vi "Send Speed Message_Conti.vi"(6 "Data":u16 format="%x", 8 "Standstill":bool, 9 "Reset":bool) -> (2 "Bit 1 Out":bool, 3 "Bit 0 Out":bool)   [LabVIEW 2015]
uses:
  Protocol State.ctl
  <vilib>/rvi/Emulation/niFpgaSctlEmulationGetInTimedLoop.vi
  <vilib>/rvi/Emulation/niFpgaProcessEmulError.vi
panel:
  out "Timer":u32
  out "Temp Data":u16
  out "State":T1
  out "Bit Count":i32
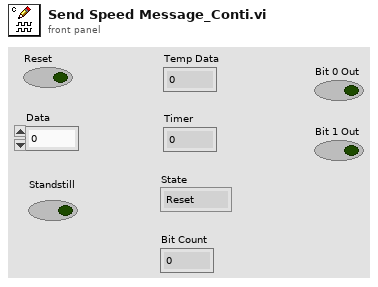
[diagram p1: front panel]
types:
  T1 = typedef "Protocol State.ctl" = enum16{"Reset", "Speed Pulse", "Delay After SP", "DP First Half", "Delay During First Half", "DP Second Half", "Delay During Second Half", "Idle"}
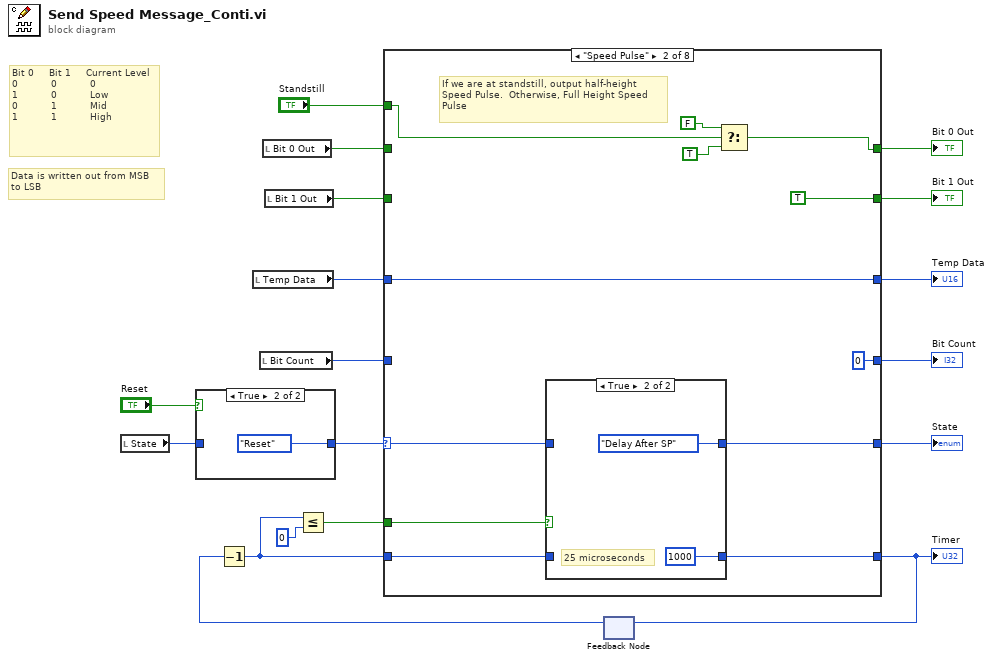
[diagram p0: block diagram]
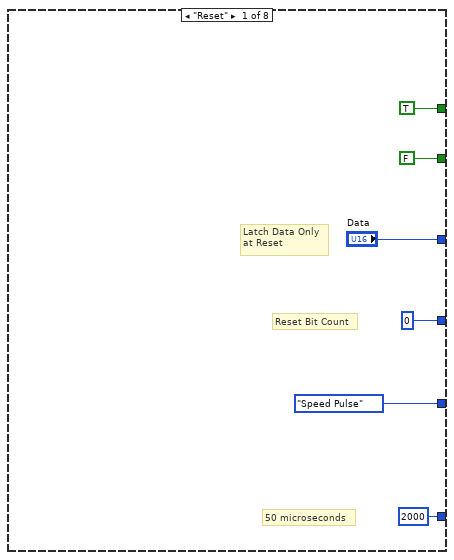
[diagram p3: hidden frame]
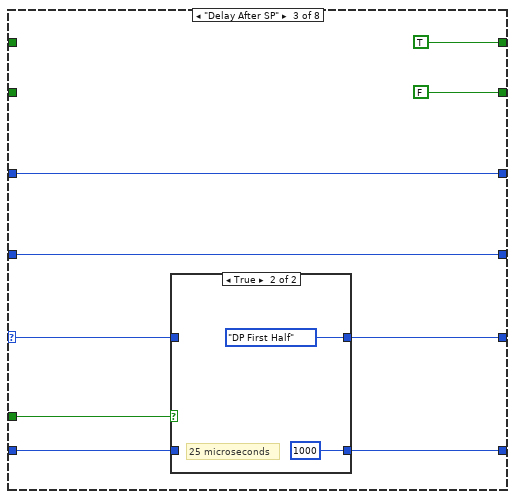
[diagram p5: hidden frame]
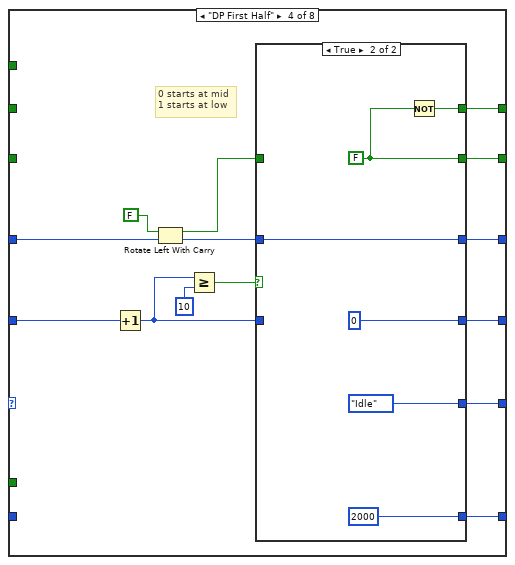
[diagram p7: hidden frame]
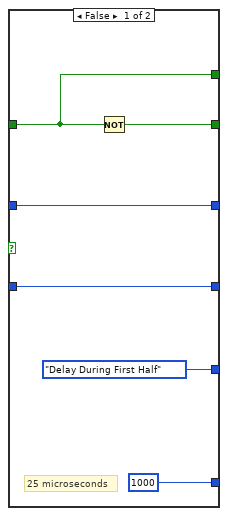
[diagram p8: hidden frame]
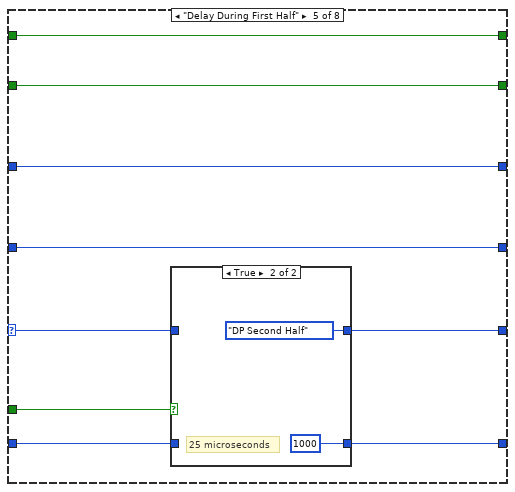
[diagram p9: hidden frame]
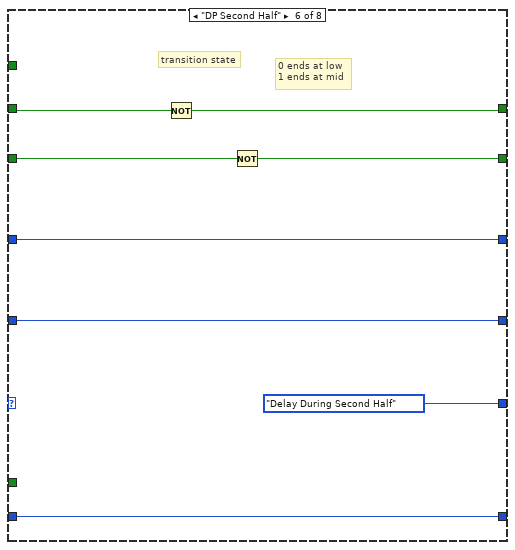
[diagram p11: hidden frame]
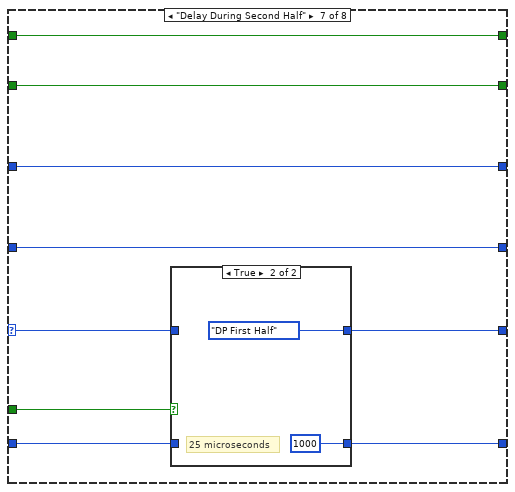
[diagram p12: hidden frame]
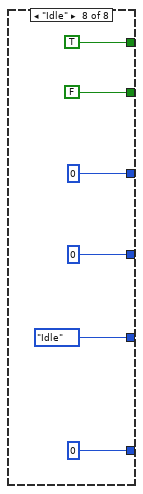
[diagram p14: hidden frame]
diagram:
  # "Data is written out from MSB\nto LSB"
  # "Bit 0     Bit 1     Current Level\n0           0           0\n1           0           Low\n0           1           Mid\n1           1           High"
  n1 = local read "State"() -> (w8:T1)
  n2 = case shown="True" "Reset" {
    tunnel: w8 -> [w19 _]
    tunnel: [w19 Protocol_State."Reset" ("State")] -> w13
    frame False {
    }
    frame True {
    }
  }
  n3 = local read "Temp Data"() -> (w6:u16)
  n4 = local read "Bit Count"() -> (w5:i32)
  n5 = local read "Bit 0 Out"() -> (w2:bool)
  n6 = local read "Bit 1 Out"() -> (w7:bool)
  n7 = feedback #1() -> (w10:u32)  [unwired: 1 in]
  n8 = Decrement(x=w10) -> (x-1=w4:u32)
  n9 = Less Or Equal?(x=w4, y=u32 0 ("x")) -> (x <= y?=w9:bool)
  n10 = case shown="\"Speed Pulse\"" w13 {
    selector: w13 -> [_ w34 w47 _ w87 _ w108 _]
    tunnel: [0 ("Bit Count") 0 ("Bit Count") w43 w68 w84 w99 w105 0 ("Bit Count")] -> w18
    tunnel: [FALSE ("carry") TRUE ("lsb carry out") FALSE ("msb carry out") w65 w83 w102 w103 FALSE ("Bit 0 Out")] -> w17
    tunnel: ["Data" w31 w44 w61 w85 w100 w106 u16 0 ("Data")] -> w16
    tunnel: [TRUE ("carry") w27 TRUE ("carry") w56 w82 w95 w104 TRUE ("carry")] -> w15
    tunnel: [Protocol_State."Speed Pulse" ("State") w33 w46 w60 w86 Protocol_State."Delay During Second Half" ("State") w107 Protocol_State."Idle" ("State")] -> w14
    tunnel: [u32 2000 ("Timer") w36 w49 w59 w89 w98 w110 u32 0 ("Timer")] -> w11
    tunnel: w4 -> [_ w35 w48 _ w88 w98 w109 _]
    tunnel: w9 -> [_ w37 w50 _ w90 _ w111 _]
    tunnel: w7 -> [_ _ _ _ w83 w97 w103 _]
    tunnel: w6 -> [_ w31 w44 w58 w85 w100 w106 _]
    tunnel: w5 -> [_ _ w43 w57 w84 w99 w105 _]
    tunnel: w2 -> [_ _ _ _ w82 w96 w104 _]
    tunnel: "Standstill" -> [_ w30 _ _ _ _ _ _]
    frame "Reset" {
      # "Latch Data Only\nat Reset"
      # "50 microseconds"
      # "Reset Bit Count"
    }
    frame "Speed Pulse" {
      # "If we are at standstill, output half-height\nSpeed Pulse.  Otherwise, Full Height Speed\nPulse"
      n11 = case shown="True" w37 {
        tunnel: [w40 u32 1000 ("Timer")] -> w36
        tunnel: w35 -> [w40 _]
        tunnel: w34 -> [w39 _]
        tunnel: [w39 Protocol_State."Delay After SP" ("State")] -> w33
        frame False {
        }
        frame True {
          # "25 microseconds"
        }
      }
      n12 = Select(t=FALSE, s=w30, f=TRUE) -> (s? t:f=w27:bool)
    }
    frame "Delay After SP" {
      n13 = case shown="True" w50 {
        tunnel: [w53 u32 1000 ("Timer")] -> w49
        tunnel: w48 -> [w53 _]
        tunnel: w47 -> [w52 _]
        tunnel: [w52 Protocol_State."DP First Half" ("State")] -> w46
        frame False {
        }
        frame True {
          # "25 microseconds"
        }
      }
    }
    frame "DP First Half" {
      # "0 starts at mid \n1 starts at low"
      n14 = Increment(x=w57) -> (x+1=w62:i32)
      n15 = Rotate Left With Carry(2:w58, 3:FALSE ("carry")) -> (0:w63:u16, 1:w66:bool)
      n16 = Greater Or Equal?(x=w62, y=10 ("x")) -> (x >= y?=w69:bool)
      n17 = case shown="True" w69 {
        tunnel: [w75 0] -> w68
        tunnel: w62 -> [w75 _]
        tunnel: [w71 w77] -> w65
        tunnel: w66 -> [w70 _]
        tunnel: w63 -> [w74 w80]
        tunnel: [w74 w80] -> w61
        tunnel: [Protocol_State."Delay During First Half" ("State") Protocol_State."Idle" ("State")] -> w60
        tunnel: [u32 1000 ("Timer") u32 2000 ("Timer")] -> w59
        tunnel: [w70 w76] -> w56
        frame False {
          # "25 microseconds"
          n18 = Not(x=w70) -> (.not. x?=w71:bool)
        }
        frame True {
          w77 = FALSE ("msb carry out")
          n19 = Not(x=w77) -> (.not. x?=w76:bool)
        }
      }
    }
    frame "Delay During First Half" {
      n20 = case shown="True" w90 {
        tunnel: [w92 u32 1000 ("Timer")] -> w89
        tunnel: w88 -> [w92 _]
        tunnel: w87 -> [w91 _]
        tunnel: [w91 Protocol_State."DP Second Half" ("State")] -> w86
        frame False {
        }
        frame True {
          # "25 microseconds"
        }
      }
    }
    frame "DP Second Half" {
      # "0 ends at low \n1 ends at mid"
      # "transition state"
      n21 = Not(x=w96) -> (.not. x?=w95:bool)
      n22 = Not(x=w97) -> (.not. x?=w102:bool)
    }
    frame "Delay During Second Half" {
      n23 = case shown="True" w111 {
        tunnel: [w113 u32 1000 ("Timer")] -> w110
        tunnel: w109 -> [w113 _]
        tunnel: w108 -> [w112 _]
        tunnel: [w112 Protocol_State."DP First Half" ("State")] -> w107
        frame False {
        }
        frame True {
          # "25 microseconds"
        }
      }
    }
    frame "Idle" {
    }
  }
  "Bit Count" <- w18
  "Bit 1 Out" <- w17
  "State" <- w14
  "Temp Data" <- w16
  "Timer" <- w11
  "Bit 0 Out" <- w15
  n24 = feedback-in #1(w11) -> ()
